vi "Get LVCompare Options.vi"(8 "error in":errorcluster) -> (0 "error out":errorcluster, 1 "TimeOut on Error":i32=250, 2 "Retries":i32=10, 3 "compare options":T1={"VI Attributes"=TRUE, "Front Panel"=TRUE, "FP position/size"=TRUE, "Block Diagram"=TRUE, "BD cosmetic"=TRUE, "BD position/size"=TRUE})   [LabVIEW 2020, in "Approval Tests.lvlib"]
uses:
  Approval Tests.lvlib
  LVCompare Options.ctl
  Global.vi
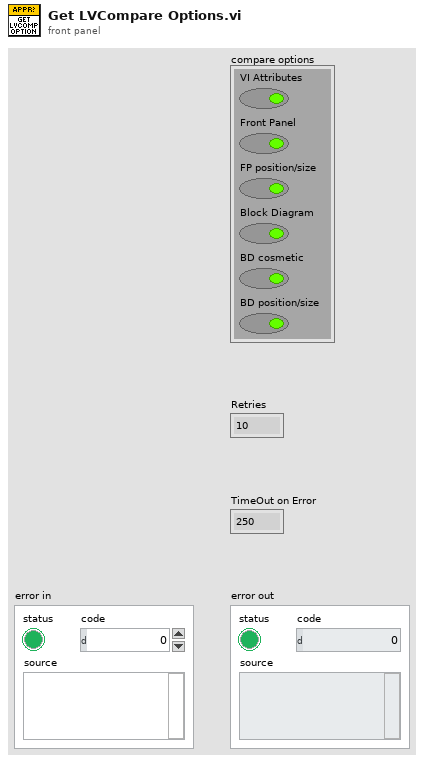
[diagram p1: front panel]
types:
  T1 = typedef "Approval Tests.lvlib/LVCompare Options.ctl" = cluster{"VI Attributes":bool, "Front Panel":bool, "FP position/size":bool, "Block Diagram":bool, "BD cosmetic":bool, "BD position/size":bool}
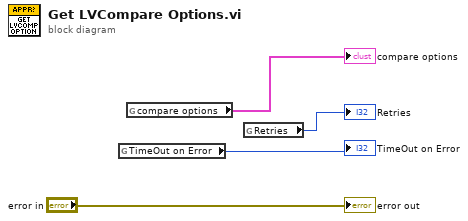
[diagram p0: block diagram]
diagram:
  n1 = global read "Global.vi" "TimeOut on Error"() -> (→"TimeOut on Error":i32)
  n2 = global read "Global.vi" "compare options"() -> (→"compare options":T1)
  n3 = global read "Global.vi" "Retries"() -> (→"Retries":i32)
  "error out" <- "error in"
